vi "Generate Nodes Item.vi"(8 "error in (no error)":errorcluster, 9 "Tree Item In":T1, 10 "Root Tag In":string, 11 "Tree Data Folder in":refnum<class "Tree Data Folder.lvclass">) -> (0 "error out":errorcluster, 1 "Nodes Item Out":T1[](array[typedef]), 3 "Tree Data Folder out":refnum<class "Tree Data Folder.lvclass">)   [LabVIEW 2022 SP3, in "Tree Data Folder.lvclass"]
uses:
  Tree Data Folder.lvclass
  Tree/Type Def/Tree Item.ctl
  Composite Tree Data/Composite Tree Data.lvclass
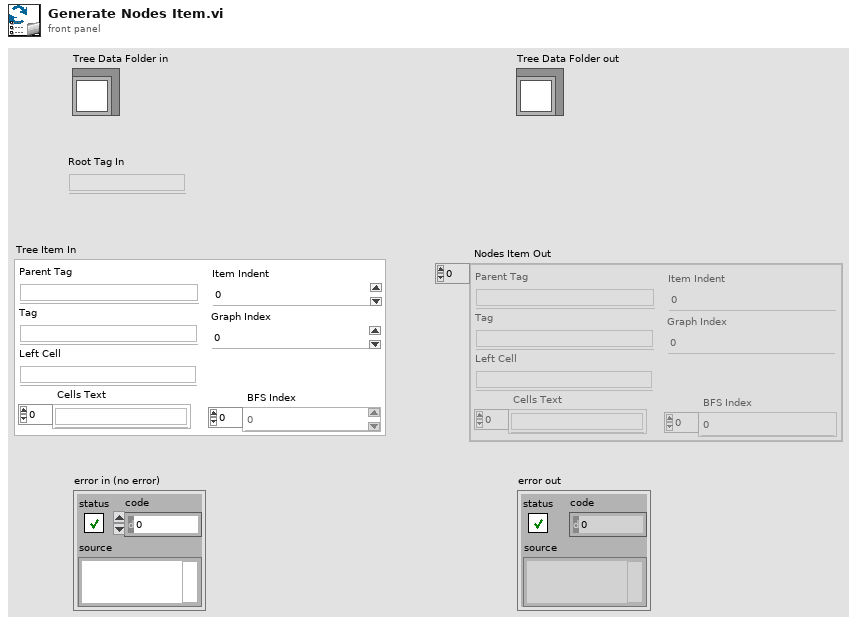
[diagram p1: front panel]
types:
  T1 = typedef "Tree Item.ctl" = cluster{"Parent Tag":string, "Tag":string, "Left Cell":string, "Cells Text":string[], "BFS Index":i32[], "Graph Index":i32, "Item Indent":i32}
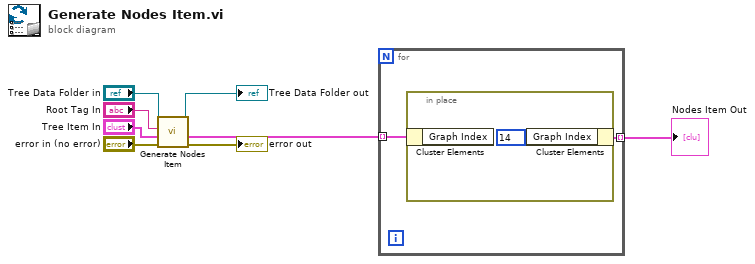
[diagram p0: block diagram]
diagram:
  n1 = call-parent "Generate Nodes Item.vi"("error in (no error)"="error in (no error)", "Tree Item In"="Tree Item In", "Root Tag In"="Root Tag In", "Composite Tree Data in"="Tree Data Folder in") -> ("error out"=→"error out":errorcluster, "Nodes Item Out"=w2:T1[], "Composite Tree Data out"=→"Tree Data Folder out":refnum<class "Tree Data Folder.lvclass">)  [unwired: 5 in]
  n2 = for {
    tunnel: w2 -> [w10] mode=indexing
    tunnel: [w9] -> w1 mode=indexing
    n3 = in-place {
      n4 = in-place-cluster #1(w10) -> ()  [unwired: 1 out]
      n5 = in-place-cluster #1("Graph Index"=14) -> (w9:T1)
    }
  }
  "Nodes Item Out" <- w1
